vi "Wait On Timer.vi"(4 "error in (no error)":errorcluster, 5 "timer value to wait for in seconds":dbl format="%.3f", 7 "timer":T1) -> (0 "error out":errorcluster, 1 "timed out":bool, 3 "timer out":T1)   [LabVIEW 2011]
doc: "Waits for a timer to be stopped, or to timeout.\n\n© Copyright 1999\nCal-Bay Systems, Inc.\nwritten by James Kring"
uses:
  Timer Refnum.ctl
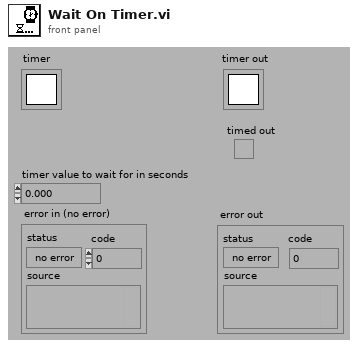
[diagram p1: front panel]
types:
  T1 = typedef "Timer Refnum.ctl" = refnum<k1>
  T2 = enum16{"open ref", "lookup ref", "close ref", "test ref", "start", "stop", "wait", "reset", "increment # waiting", "decrement #waiting"}
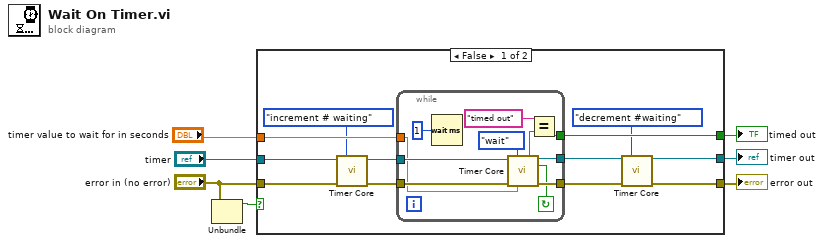
[diagram p0: block diagram]
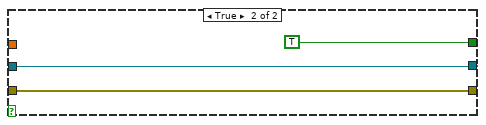
[diagram p2: hidden frame]
diagram:
  n1 = Unbundle("error in (no error)") -> ("status"=w2:bool)  [unwired: 2 out]
  n2 = case shown="False" w2 {
    tunnel: [w9 w33] -> w7
    tunnel: "error in (no error)" -> [w16 w33]
    tunnel: [w19 TRUE ("timed out")] -> w6
    tunnel: "timer" -> [w17 w32]
    tunnel: [w10 w32] -> w4
    tunnel: "timer value to wait for in seconds" -> [w18 _]
    frame False {
      n3 = call "Timer Core.vi"("timer"=w17, "function"=T2."increment # waiting", "error in (no error)"=w16) -> ("timer out"=w14:T1, "error out"=w15:errorcluster)  [unwired: 6 in, 5 out]
      n4 = while {
        tunnel: w18 -> [w21]
        tunnel: [w27] -> w19
        tunnel: w14 -> [w23]
        tunnel: [w30] -> w12
        tunnel: w15 -> [w22]
        tunnel: [w28] -> w11
        stop <- w26 continue-if-true
        n5 = Wait (ms)(milliseconds to wait=u32 1) -> ()  [unwired: 1 out]
        n6 = call "Timer Core.vi"("timer"=w23, "function"=T2."wait", "error in (no error)"=w22, "Wait timeout [sec]"=w21) -> ("timer out"=w30:T1, "Keep Waiting"=w26:bool, "message out"=w24:string, "error out"=w28:errorcluster)  [unwired: 5 in, 3 out]
        n7 = Equal?(x="timed out" ("y"), y=w24) -> (x = y?=w27:bool)
      }
      n8 = call "Timer Core.vi"("timer"=w12, "function"=T2."decrement #waiting", "error in (no error)"=w11) -> ("timer out"=w10:T1, "error out"=w9:errorcluster)  [unwired: 6 in, 5 out]
    }
    frame True {
    }
  }
  "timer out" <- w4
  "error out" <- w7
  "timed out" <- w6
